vi "scan2d_acquire_new_data.vi"(8 "error in (no error)":errorcluster, 11 "scan_2d in":refnum<class "scan_2d.lvclass">) -> (0 "error out":errorcluster, 3 "scan_2d out":refnum<class "scan_2d.lvclass">)   [LabVIEW 2015, in "scan_2d.lvclass"]
uses:
  scan_2d.lvclass
  scan_2d.lvclass/scan_2d.ctl
  Detector_Class/detector/detector.lvclass
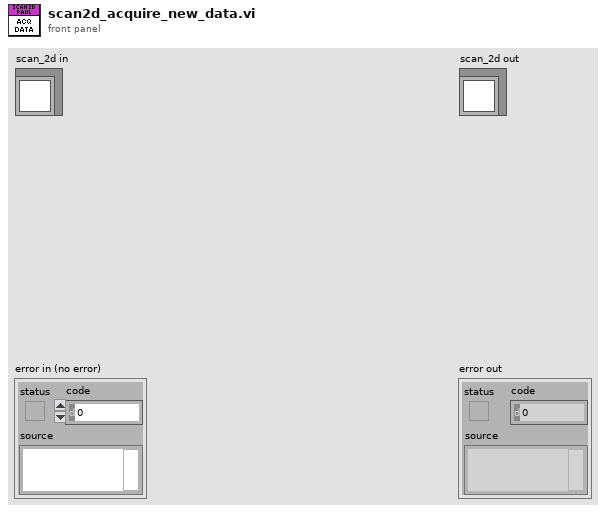
[diagram p1: front panel]
types:
  T1 = typedef "detector_data_tdef.ctl" = cluster{"data_array":dbl[][][], "data_size":cluster{"X":i32, "Y":i32, "Z":i32}}
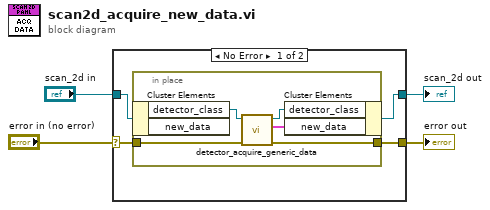
[diagram p0: block diagram]
diagram:
  n1 = case shown="No Error" "error in (no error)" {
    selector: "error in (no error)" -> [w7 w15]
    tunnel: [w6 w15] -> w3
    tunnel: [w5 w14] -> w1
    tunnel: "scan_2d in" -> [w8 w14]
    frame No Error {
      n2 = in-place {
        in-place-border: w7 -> [w11]
        in-place-border: [w10] -> w6
        n3 = in-place-cluster #1(w8) -> ("detector_class"=w13:refnum<class "detector.lvclass">)  [unwired: 1 out]
        n4 = call-dynamic "detector_acquire_generic_data.vi"("error in (no error)"=w11, "detector in"=w13) -> ("error out"=w10:errorcluster, "detector_output"=w9:T1, "detector out"=w12:refnum<class "detector.lvclass">)  [unwired: 7 in]
        n5 = in-place-cluster #1("detector_class"=w12, "new_data"=w9) -> (w5:refnum<class "scan_2d.lvclass">)
      }
    }
    frame Error {
    }
  }
  "error out" <- w3
  "scan_2d out" <- w1
